vi "1_VI_LIDAR_CAL2.vi"(11 "Analog input":dbl=0.745849533 format="%0.2f") -> (3 "LidarDistance":dbl=757.2004722400102)   [LabVIEW 2019]
uses:
  <vilib>/ptbypt/NI_PtbyPt.lvlib
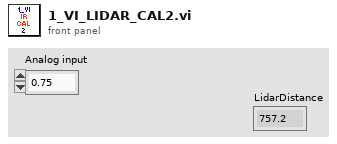
[diagram p1: front panel]
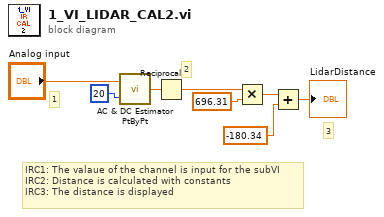
[diagram p0: block diagram]
diagram:
  # "3"
  # "2"
  # "1"
  # "IRC1: The valaue of the channel is input for the subVI\nIRC2: Distance is calculated with constants\nIRC3: The distance is displayed"
  n1 = call <vilib>:"AC & DC Estimator PtByPt.vi"("signal"="Analog input", "sample length"=20) -> ("DC estimate (V)"=w7:dbl)  [unwired: 1 in, 2 out]
  n2 = Reciprocal(x=w7) -> (1/x=w6:dbl)
  n3 = Multiply(x=w6, y=696.31) -> (x*y=w5:dbl)
  n4 = Add(x=w5, y=-180.34) -> (x+y=→"LidarDistance":dbl)
